vi "Set Trigger Sweep Signal.vi"(6 "Delay (0.0)":dbl format="%.2f", 7 "Trigger Level (0: Low )":u16(ring) items=["Low", "High"], 8 "Error In (no error)":errorcluster, 9 "Trigger Scope (0: All Channels )":u16(ring) items=["All Channels", "Current Chann."], 10 "Source (0: Immediate)":u16(ring) items=["Immediate", "External", "Manual"], 11 "VISA session":refnum<visa-resource-name>) -> (0 "Error Out":errorcluster, 3 "dup VISA session":refnum<visa-resource-name>)   [LabVIEW 2018, in "Agilent PNA Series.lvlib"]
doc: "This VI sets the source of the sweep trigger signal."
uses:
  Agilent PNA Series.lvlib
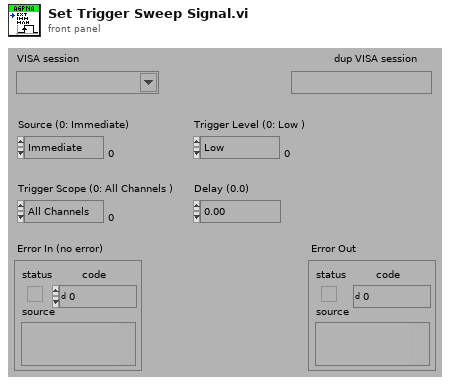
[diagram p1: front panel]
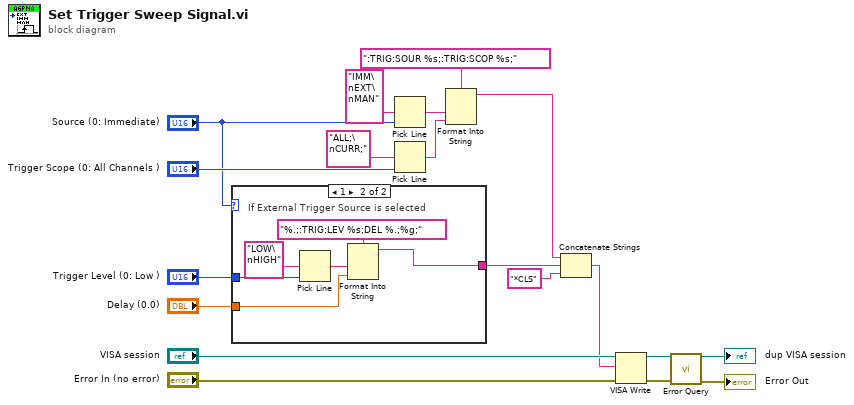
[diagram p0: block diagram]
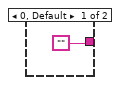
[diagram p2: hidden frame]
diagram:
  n1 = case shown="1" "Source (0: Immediate)" {
    tunnel: "Trigger Level (0: Low )" -> [_ w25]
    tunnel: "Delay (0.0)" -> [_ w21]
    tunnel: ["" w23] -> w10
    frame 0, Default {
    }
    frame 1 {
      # "If External Trigger Source is selected"
      n2 = Pick Line(multi-line string="LOW\nHIGH", line index=w25) -> (output string=w22:string)  [unwired: 1 in]
      n3 = Format Into String(format string="%.;:TRIG:LEV %s;DEL %.;%g;", w22, w21) -> (resulting string=w23:string)  [unwired: 2 in, 1 out]
    }
  }
  n4 = Pick Line(multi-line string="IMM\nEXT\nMAN", line index="Source (0: Immediate)") -> (output string=w9:string)  [unwired: 1 in]
  n5 = Pick Line(multi-line string="ALL;\nCURR;", line index="Trigger Scope (0: All Channels )") -> (output string=w8:string)  [unwired: 1 in]
  n6 = Format Into String(format string=":TRIG:SOUR %s;:TRIG:SCOP %s;", w9, w8) -> (resulting string=w7:string)  [unwired: 2 in, 1 out]
  n7 = Concatenate Strings(w7, w10, "*CLS" ("string")) -> (w16:string)
  n8 = VISA Write(VISA resource name="VISA session", write buffer=w16, error in (no error)="Error In (no error)") -> (VISA resource name out=w4:refnum<visa-resource-name>, error out=w3:errorcluster)  [unwired: 1 out]
  n9 = call "Error Query.vi"("VISA Resource Name"=w4, "error in (no error)"=w3) -> ("VISA Resource Name Out"=→"dup VISA session":refnum<visa-resource-name>, "error out"=→"Error Out":errorcluster)  [unwired: 10 in, 2 out]
